vi "rad_NI-Auth Login Dialog.vi"(8 "error in (no error)":errorcluster, 11 "Target Address":string="10.0.19.46") -> (0 "error out":errorcluster, 1 "Cancelled":bool, 2 "Password Out":string, 3 "session out":refnum<k21>)   [LabVIEW 2021]
uses:
  <vilib>/nisyscfg/Close (System).vi
  <vilib>/nisyscfg/nisyscfg.lvlib
panel:
  out "Target":string
  in  "Cancel":bool
  in  "RetireveImg":bool
  in  "Password":string
  # "Permission required for"
  # "User Name: admin"
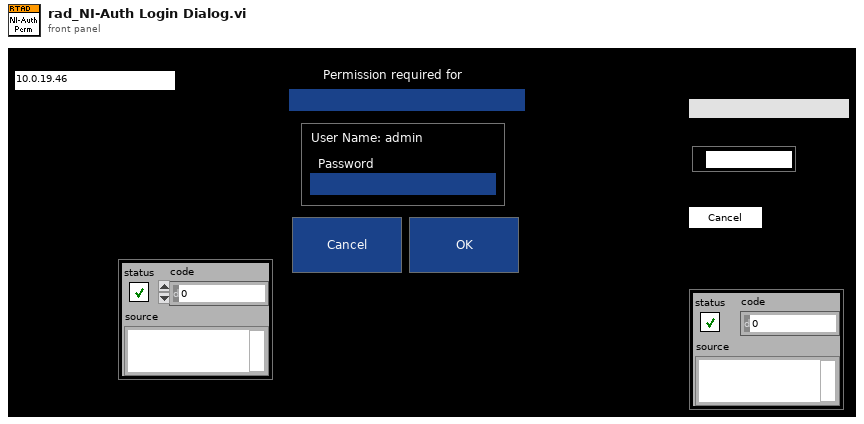
[diagram p1: front panel]
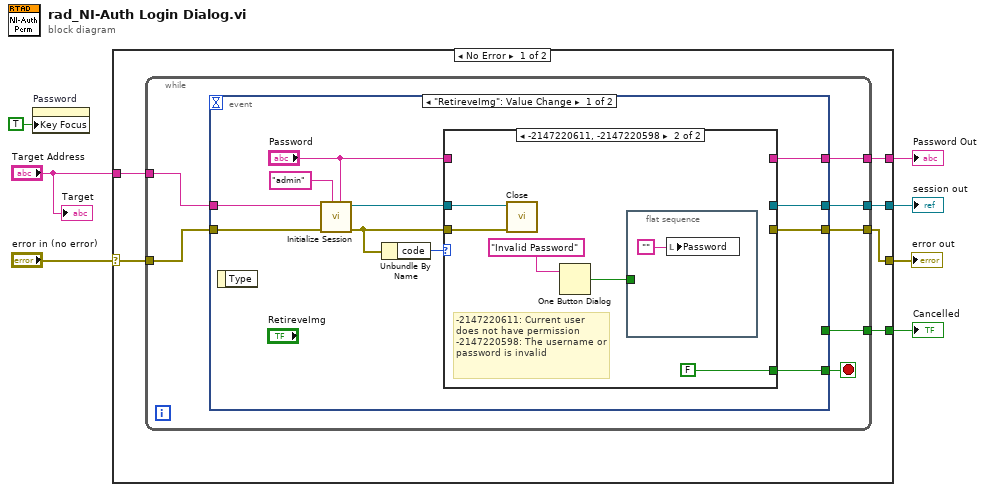
[diagram p0: block diagram]
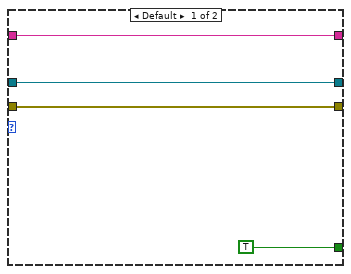
[diagram p2: hidden frame]
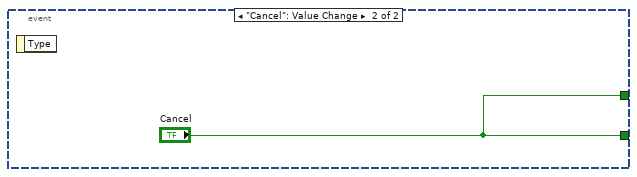
[diagram p3: hidden frame]
diagram:
  n1 = property on="Password" class="Str"("Key Focus"=TRUE) -> ()  [unwired: 2 in, 2 out]
  n2 = case shown="No Error" "error in (no error)" {
    selector: "error in (no error)" -> [w8 w43]
    tunnel: "Target Address" -> [w13 _]
    tunnel: [w12 w43] -> w7
    tunnel: [w11 _] -> w6
    tunnel: [w10 _] -> w5
    tunnel: [w9 _] -> w4
    frame No Error {
      n3 = while {
        tunnel: w13 -> [w20]
        tunnel: [w18] -> w12
        tunnel: [w17] -> w11
        tunnel: [w16] -> w10
        tunnel: [w15] -> w9
        tunnel: w8 -> [w14]
        stop <- w19 stop-if-true
        n4 = event shown="[0] \"RetireveImg\": Value Change" {
          selector: _ -> [_ _]
          dyn-events: _ -> [_ _]
          timeout: _ -> [_ _]
          tunnel: w20 -> [w30 _]
          tunnel: [w28 "Cancel"] -> w19
          tunnel: [w26 _] -> w18
          tunnel: [w24 _] -> w17
          tunnel: [w22 _] -> w16
          tunnel: [_ "Cancel"] -> w15
          tunnel: w14 -> [w21 _]
          event "RetireveImg": Value Change {
            n5 = event-data() -> ()  [unwired: 1 in, 1 out]
            n6 = call <vilib>:"Initialize Session.vi"("Password"="Password", "User Name"="admin" ("user name"), "error in (no error)"=w21, "Target (localhost)"=w30) -> ("error out"=w27:errorcluster, "Session out"=w23:refnum<k21>)  [unwired: 6 in]
            n7 = Unbundle By Name(w27) -> ("code"=w29:i32)
            n8 = case shown="-2147220611, -2147220598" w29 {
              tunnel: [TRUE FALSE] -> w28
              tunnel: w27 -> [w35 w37]
              tunnel: [w35 _] -> w26
              tunnel: "Password" -> [w34 _]
              tunnel: [w34 _] -> w24
              tunnel: w23 -> [w32 w38]
              tunnel: [w32 _] -> w22
              frame Default {
              }
              frame -2147220611, -2147220598 {
                # "-2147220611: Current user does not have permission\n-2147220598: The username or password is invalid"
                n9 = call-poly <vilib>:"Close.vi"("error in (no error)"=w37, "Session in"=w38) -> ()  [unwired: 9 in, 1 out]
                n10 = One Button Dialog(message="Invalid Password") -> (true=w36:bool)  [unwired: 1 in]
                n11 = flat-sequence {
                  tunnel: w36 -> [_]
                  frame #0 {
                    n12 = local write "Password"("" ("Password:")) -> ()
                  }
                }
              }
            }
          }
          event "Cancel": Value Change {
            n13 = event-data() -> ()  [unwired: 1 in, 1 out]
          }
        }
      }
    }
    frame Error {
    }
  }
  "Password Out" <- w6
  "Cancelled" <- w4
  "error out" <- w7
  "session out" <- w5
  "Target" <- "Target Address"
